vi "DeleteCorruptComicFiles.vi"() -> ()   [LabVIEW 2022 SP3]
panel:
  out "error out":errorcluster
  out "Current Comic":string
  in  "Path":path=path "C:/data/comics/CorruptComics.txt"
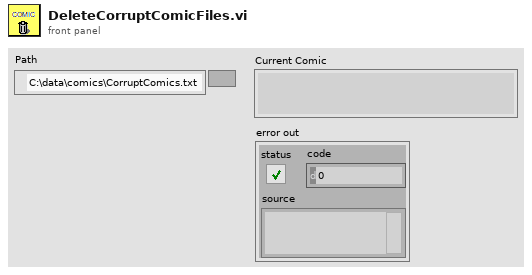
[diagram p1: front panel]
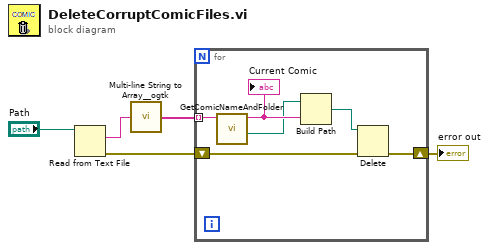
[diagram p0: block diagram]
diagram:
  n1 = Read from Text File(file (use dialog)="Path") -> (text=w4:string, error out=w3:errorcluster)  [unwired: 3 in, 2 out]
  n2 = call <userlib>:"Multi-line String to Array__ogtk.vi"("string"=w4) -> ("lines"=w2:string[])
  n3 = for {
    shift-right: [w8] -> w1
    shift-left: w3 -> [w7]
    tunnel: w2 -> [w11] mode=indexing
    n4 = call "GetComicNameAndFolder.vi"("URL"=w11) -> ("OwningFolder"=w9:path, "FileName"=w10:string)  [unwired: 9 in]
    "Current Comic" <- w10
    n5 = Build Path(base path=w9, name or relative path=w10) -> (appended path=w6:path)
    n6 = Delete(path (use dialog)=w6, error in=w7) -> (error out=w8:errorcluster)  [unwired: 3 in, 2 out]
  }
  "error out" <- w1
